vi "Initialize.vi"(7 "Serial Configuration":T1={"Baud Rate"=9600, "Parity"=0, "Data Bits"=8, "Stop Bits"=10, "Flow Control"=0} {"Flow Control" items=["None", "XON/XOFF", "RTS/CTS", "XON/XOFF & RTS/CTS", "DTR/DSR", "XON/XOFF & DTR/DSR"]; "Stop Bits" items=["1.0"=10, "1.5"=15, "2.0"=20]; "Data Bits" items=["7"=7, "8"=8]; "Parity" items=["None", "Odd", "Even", "Mark", "Space"]; "Baud Rate" items=["300"=300, "600"=600, "1200"=1200, "2400"=2400, "4800"=4800, "9600"=9600, "19200"=19200]}, 8 "error in":errorcluster, 11 "VISA resource name":refnum<visa-resource-name>) -> (0 "error out":errorcluster, 3 "VISA resource name out":refnum<visa-resource-name>)   [LabVIEW 2020, in "IT-M3400.lvlib"]
doc: "Establishes communication with the instrument and optionally performs an instrument identification query and/or an instrument reset. It also places the instrument in a default state needed for other instrument driver operations. Therefore, call this VI before calling other instrument driver VIs for this instrument. Generally, you need to call the <b>Initialize</b> VI only once at the beginning of an application."
uses:
  <instrlib>/IT-M3400/IT-M3400.lvlib
panel:
  # "EDIT: Change control description to remove example text for buses not supported."
  # "EDIT: Serial settings must match those on the physical instrument.  Review user's manual to determine the correct Flow Control protocol for the instrument.  \"None\" is the least robust option for this setting, and could lead to unreliable data transmission."
  # "EDIT: If your instrument does not support ID query or Reset, remove the ID Query or Reset control from the front panel and delete the case structure with the ID Query or Reset code from the block diagram."
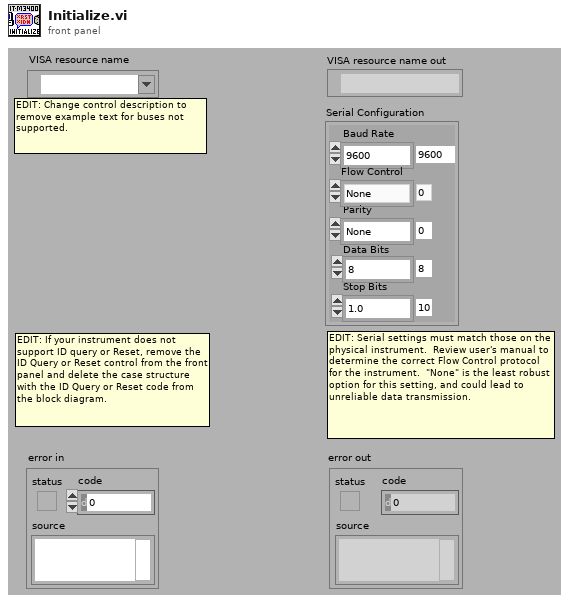
[diagram p1: front panel]
types:
  T1 = cluster{"Baud Rate":u32, "Parity":u16, "Data Bits":u16, "Stop Bits":u16, "Flow Control":u16}
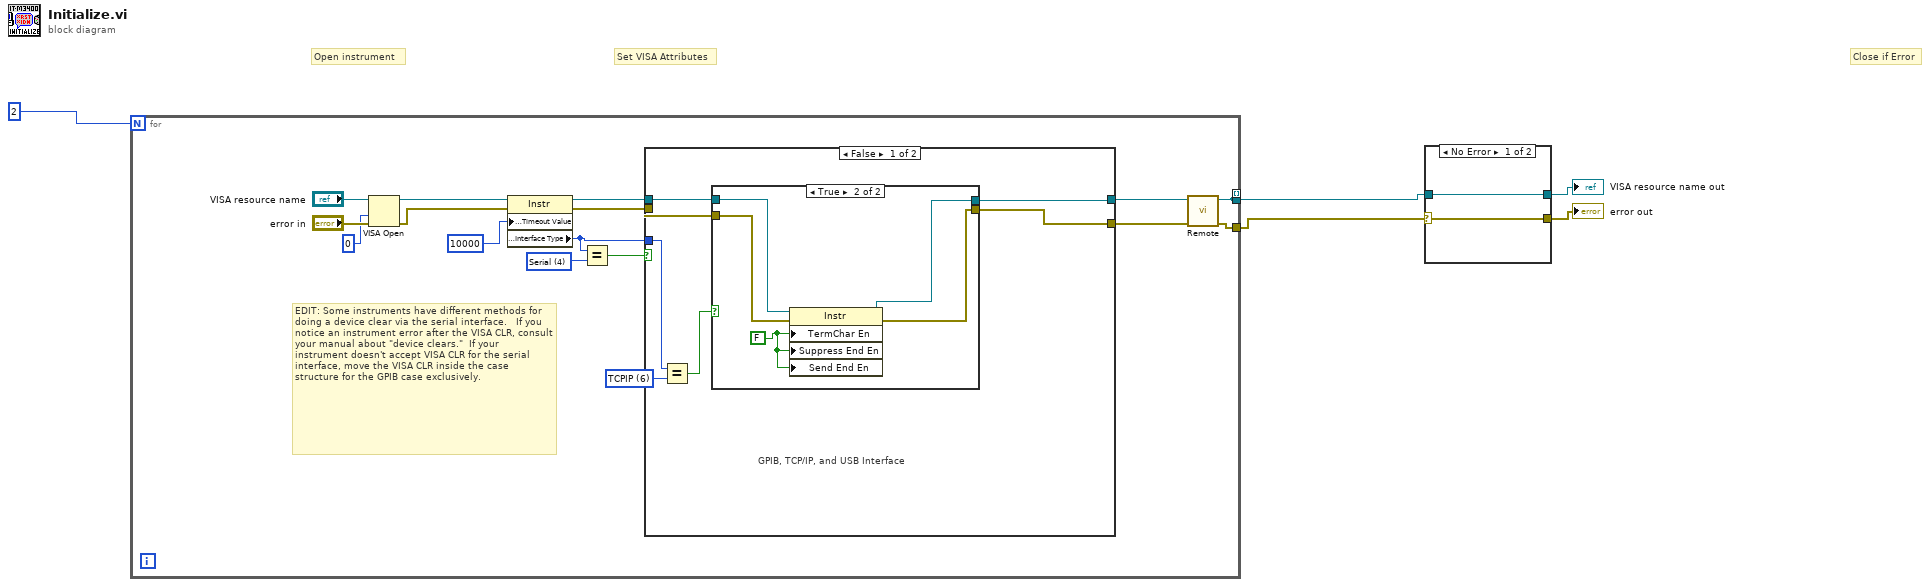
[diagram p0: block diagram]
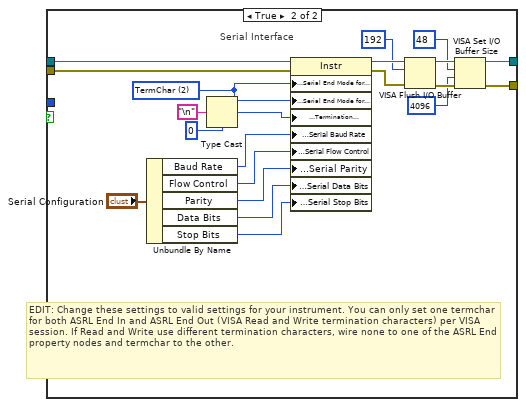
[diagram p3: hidden frame]
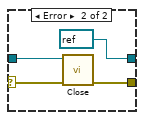
[diagram p4: hidden frame]
diagram:
  # "Set VISA Attributes"
  # "Close if Error"
  # "Open instrument"
  n1 = for {
    N: 2 -> [_]
    tunnel: [w6] -> w2
    tunnel: [w10] -> w1
    tunnel: [w6] -> _ mode=indexing
    w15 = u16 4 items=["GPIB"=1, "VXI"=2, "GPIB-VXI"=3, "Serial"=4, "PXI"=5, "TCPIP"=6, "USB"=7] ("Interface Information:Interface Type")
    # "EDIT: Some instruments have different methods for doing a device clear via the serial interface.   If you notice an instrument error after the VISA CLR, consult your manual about \"device clears.\"  If your instrument doesn't accept VISA CLR for the serial interface, move the VISA CLR inside the case  structure for the GPIB case exclusively."
    n2 = VISA Open(access mode=u32 0, error in (no error)="error in", VISA resource name="VISA resource name") -> (VISA resource name=w8:refnum<visa-resource-name>, error out=w7:errorcluster)  [unwired: 2 in]
    n3 = property class="Instr"(reference=w8, error in=w7, "General Settings:Timeout Value"=u32 10000) -> (reference out=w17:refnum<visa-resource-name>, error out=w16:errorcluster, "Interface Information:Interface Type"=w13:u16)
    n4 = Equal?(x=w13, y=w15) -> (x = y?=w9:bool)
    n5 = case shown="False" w9 {
      tunnel: [w22 w52] -> w12
      tunnel: [w21 w49] -> w11
      tunnel: w17 -> [w24 w54]
      tunnel: w16 -> [w23 w55]
      tunnel: w13 -> [w25 _]
      frame False {
        w26 = u16 6 items=["GPIB"=1, "VXI"=2, "GPIB-VXI"=3, "Serial"=4, "PXI"=5, "TCPIP"=6, "USB"=7] ("Interface Information:Interface Type")
        # "GPIB, TCP/IP, and USB Interface"
        n6 = Equal?(x=w25, y=w26) -> (x = y?=w27:bool)
        n7 = case shown="True" w27 {
          tunnel: [w29 w34] -> w22
          tunnel: [w28 w33] -> w21
          tunnel: w24 -> [w29 w32]
          tunnel: w23 -> [w28 w31]
          frame False {
          }
          frame True {
            w30 = FALSE
            n8 = property class="Instr"(reference=w32, error in=w31, "TermChar En"=w30, "Suppress End En"=w30, "Send End En"=w30) -> (reference out=w34:refnum<visa-resource-name>, error out=w33:errorcluster)
          }
        }
      }
      frame True {
        w42 = u16 2 items=["None", "LastBit", "TermChar"] ("Serial Settings:Serial End Mode for Reads")
        # "EDIT: Change these settings to valid settings for your instrument. You can only set one termchar for both ASRL End In and ASRL End Out (VISA Read and Write termination characters) per VISA session. If Read and Write use different termination characters, wire none to one of the ASRL End property nodes and termchar to the other."
        # "Serial Interface"
        n9 = Unbundle By Name("Serial Configuration") -> ("Baud Rate"=w40:u32, "Flow Control"=w36:u16, "Parity"=w38:u16, "Data Bits"=w39:u16, "Stop Bits"=w35:u16)
        n10 = Type Cast(type=u8 0, x="\n" ("Line Feed Constant")) -> (*(type *) &x=w41:u8)
        n11 = property class="Instr"(reference=w54, error in=w55, "Serial Settings:Serial End Mode for Reads"=w42, "Serial Settings:Serial End Mode for Writes"=w42, "Message Based Settings:Termination Character"=w41, "Serial Settings:Serial Baud Rate"=w40, "Serial Settings:Serial Flow Control"=w36, "Serial Settings:Serial Parity"=w38, "Serial Settings:Serial Data Bits"=w39, "Serial Settings:Serial Stop Bits"=w35) -> (reference out=w48:refnum<visa-resource-name>, error out=w51:errorcluster)
        n12 = VISA Flush I/O Buffer(VISA resource name=w48, mask (16)=u16 192, error in (no error)=w51) -> (VISA resource name out=w53:refnum<visa-resource-name>, error out=w50:errorcluster)
        n13 = VISA Set I/O Buffer Size(VISA resource name=w53, mask (16)=u16 48, size (4096)=u32 4096 ("size (0)"), error in (no error)=w50) -> (VISA resource name out=w52:refnum<visa-resource-name>, error out=w49:errorcluster)
      }
    }
    n14 = call <instrlib>:"Remote.vi"("error in"=w11, "VISA resource name"=w12) -> ("error out"=w10:errorcluster, "VISA resource name out"=w6:refnum<visa-resource-name>)  [unwired: 8 in]
  }
  n15 = case shown="No Error" w1 {
    selector: w1 -> [w56 w59]
    tunnel: w2 -> [w57 w60]
    tunnel: [w57 refnum<visa-resource-name> refnum ("VISA resource name out")] -> w5
    tunnel: [w56 w61] -> w4
    frame No Error {
    }
    frame Error {
      n16 = call <instrlib>:"Close.vi"("error in"=w59, "VISA resource name"=w60) -> ("error out"=w61:errorcluster)  [unwired: 9 in]
    }
  }
  "VISA resource name out" <- w5
  "error out" <- w4
